vi "2.3.vi"() -> ()   [LabVIEW 2017]
panel:
  out "Waveform Chart":dbl(graph)
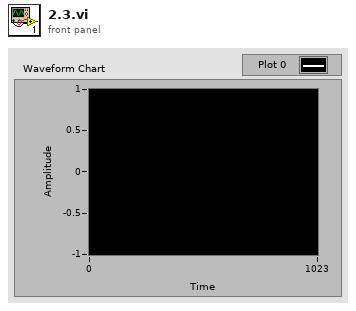
[diagram p1: front panel]
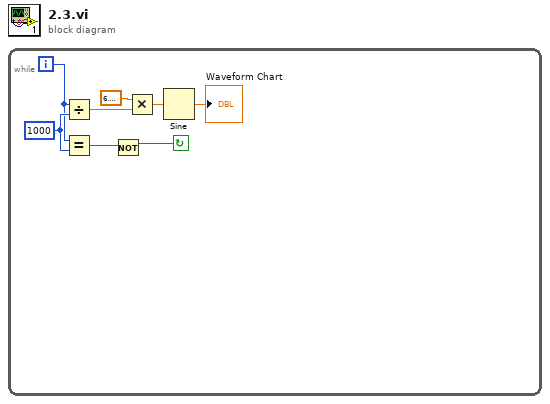
[diagram p0: block diagram]
diagram:
  n1 = while {
    i -> [w6]
    stop <- w2 continue-if-true
    w7 = 1000
    n2 = Divide(x=w6, y=w7) -> (x/y=w5:dbl)
    n3 = Equal?(x=w6, y=w7) -> (x = y?=w1:bool)
    n4 = Not(x=w1) -> (.not. x?=w2:bool)
    n5 = Multiply(x=6.283185307179586, y=w5) -> (x*y=w4:dbl)
    n6 = Sine(x=w4) -> (sin(x)=→"Waveform Chart":dbl)
  }
